vi "RequestJsonToString.vi"(8 "error in (no error)":errorcluster, 11 "Data Out":string) -> (0 "error out":errorcluster, 3 "Request":string)   [LabVIEW 2015]
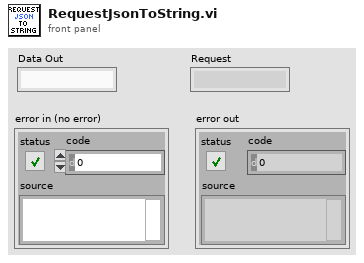
[diagram p1: front panel]
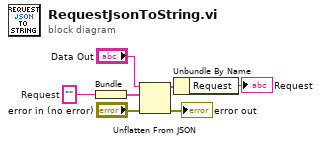
[diagram p0: block diagram]
diagram:
  w3 = ""  # Request
  n1 = Bundle("Request"=w3) -> (w4:cluster{"Request":string})  [unwired: 1 in]
  n2 = Unflatten From JSON(JSON string="Data Out", type and defaults=w4, error in (no error)="error in (no error)") -> (value=w5:cluster{"Request":string}, error out=→"error out":errorcluster)  [unwired: 4 in]
  n3 = Unbundle By Name(w5) -> ("Request"=→"Request":string)
